vi "Use_Orig_XW_Stats.vi"() -> (5 "Plug in titles":string[](array[string]), 7 "Plug in values":string[](array[string]))   [LabVIEW 2010]
uses:
  Globals/Meas_global.vi
panel:
  in  "Invert 2nd Component?":bool
  out "Array":string[](array[string])
  in  "Template Filename":path=path "/G4_2_HD/Users/paulhayden/Projects/Hong Roughness/Reclaim data.tpt"
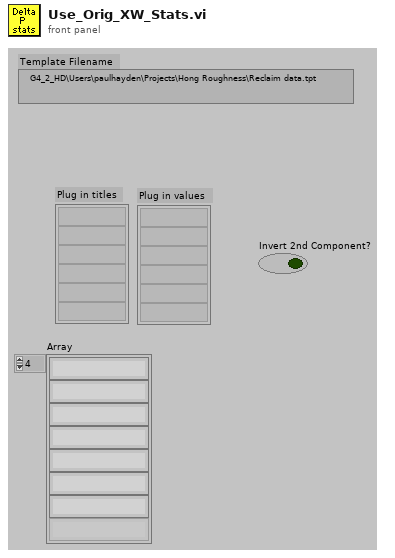
[diagram p1: front panel]
types:
  T1 = enum32{"existing file", "new file", "new or existing file", "existing dir", "new dir", "new or existing dir", "existing file (use LLBs)", "new file (use LLBs)", "new or existing file (use LLBs)", "new or existing file or directory (use LLBs)"}
  T2 = typedef "Analysis_type_cluster.ctl" = cluster{"Analysis type":T3, "Indicies":i32[], "Name":string, "Inst Array":T4, "Info index":i32}
  T3 = typedef "Analysis_type_Enum.ctl" = enum16{"Slow Response", "Fast Response", "Weighted Fast Response", "Fast FID", "Weighted Fast FID", "Cross Wire", "Weighted Cross Wire", "Weighted LDA"}
  T4 = typedef "Instrument_Array.ctl" = enum16{"PWA", "LDA", "Analogue"}
  T5 = typedef "Velocity_cluster.ctl" = cluster{"Name":string, "U":dbl, "u^2":dbl, "u^3/(u^2)^(1.5)":dbl, "u^4/(u^2)^2 -3":dbl, "% u'/U":dbl, "Mean % Err":dbl, "u^4":dbl}
  T6 = typedef "Correlation_cluster.ctl" = cluster{"U inst":string, "W inst":string, "uw":dbl, "uw/u'w'":dbl, "u^2w":dbl, "uw^2":dbl, "uw^3":dbl, "u^3w":dbl, "u^2w^2":dbl}
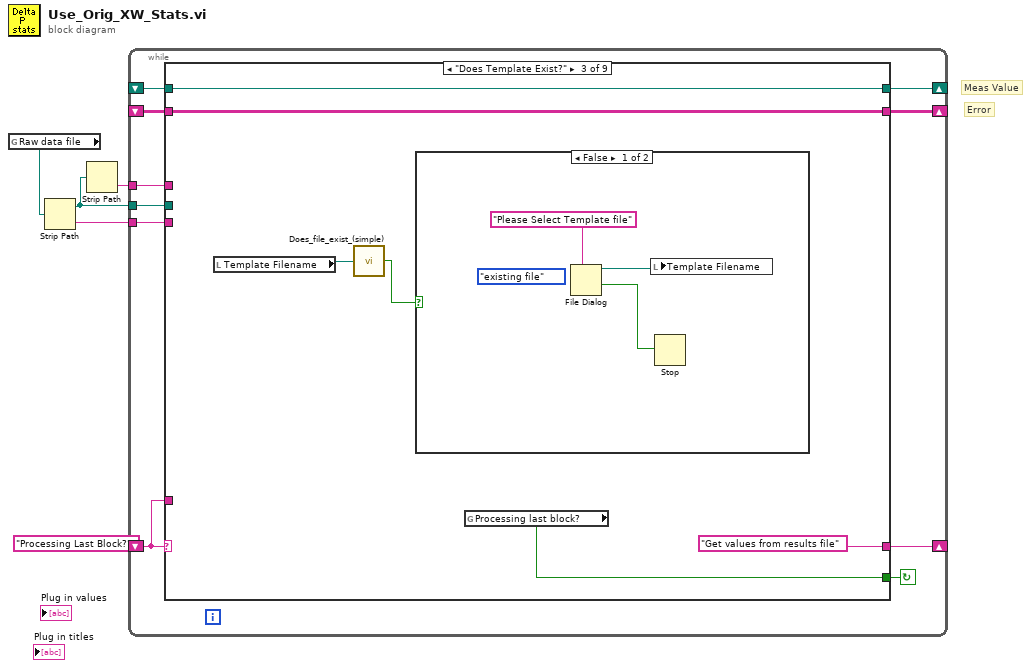
[diagram p0: block diagram]
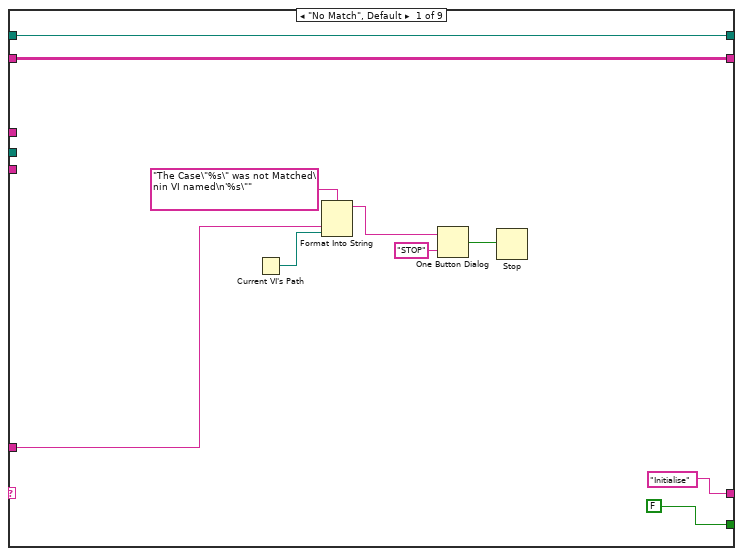
[diagram p2: hidden frame]
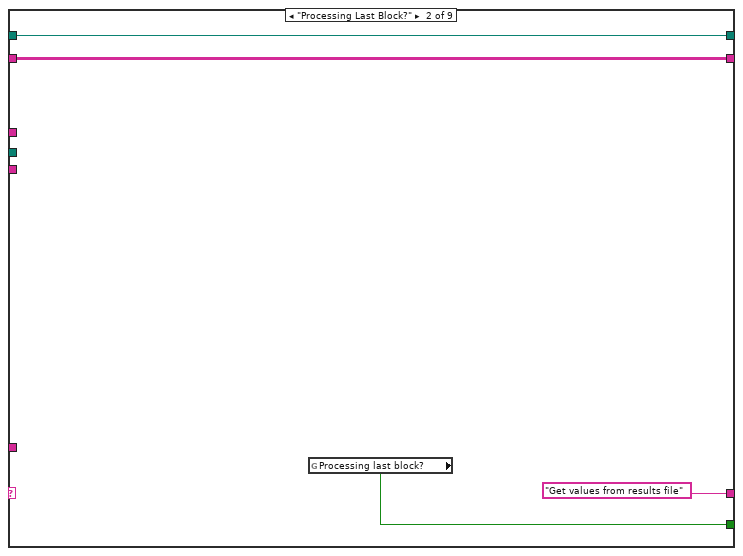
[diagram p3: hidden frame]
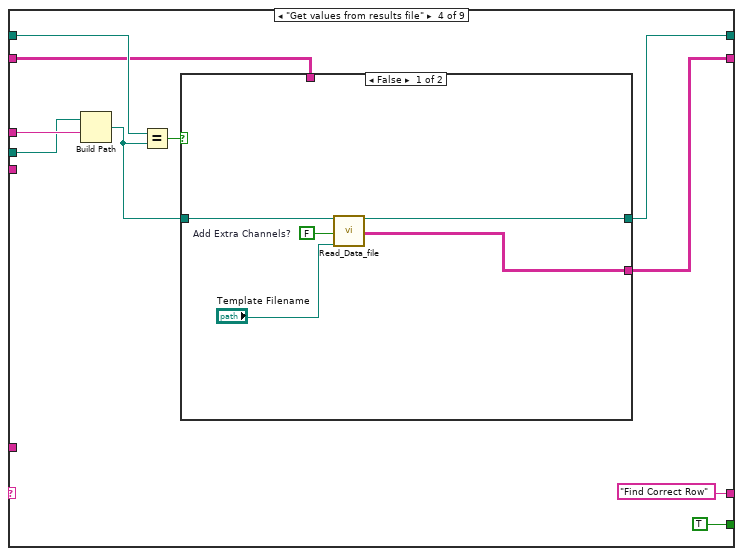
[diagram p5: hidden frame]
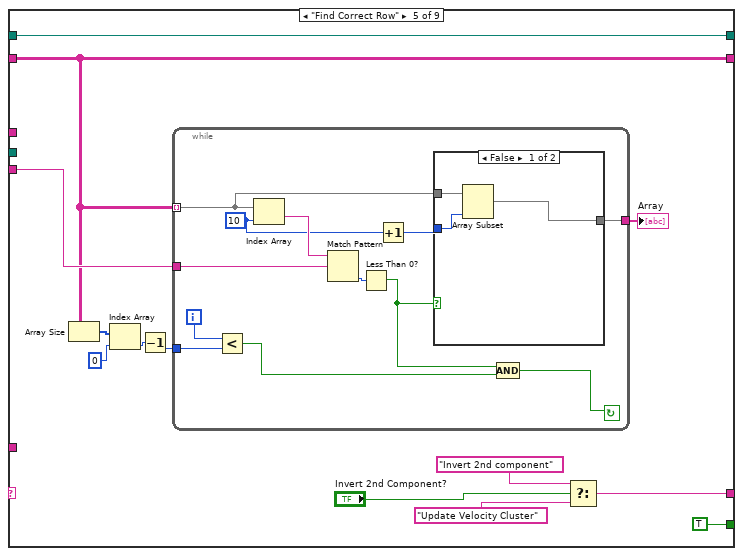
[diagram p7: hidden frame]
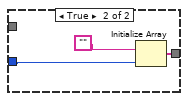
[diagram p8: hidden frame]
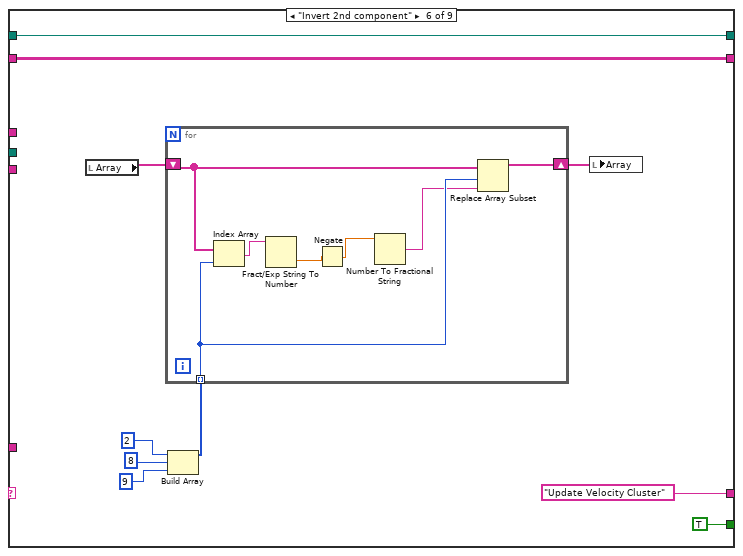
[diagram p9: hidden frame]
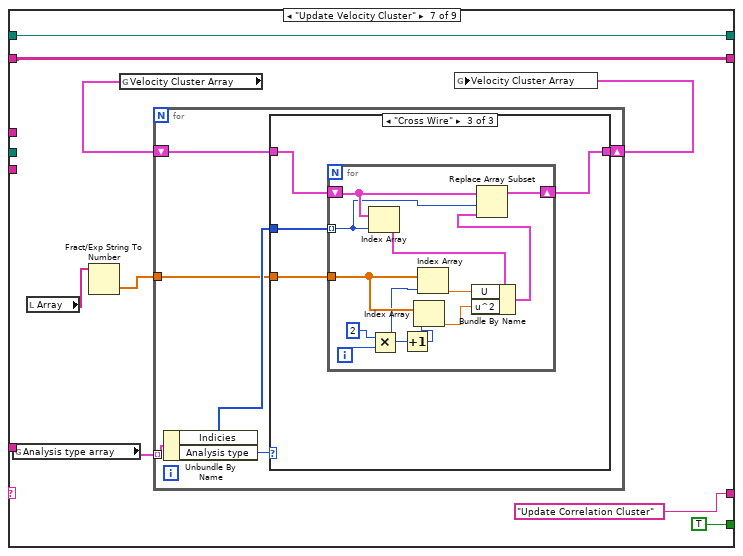
[diagram p10: hidden frame]
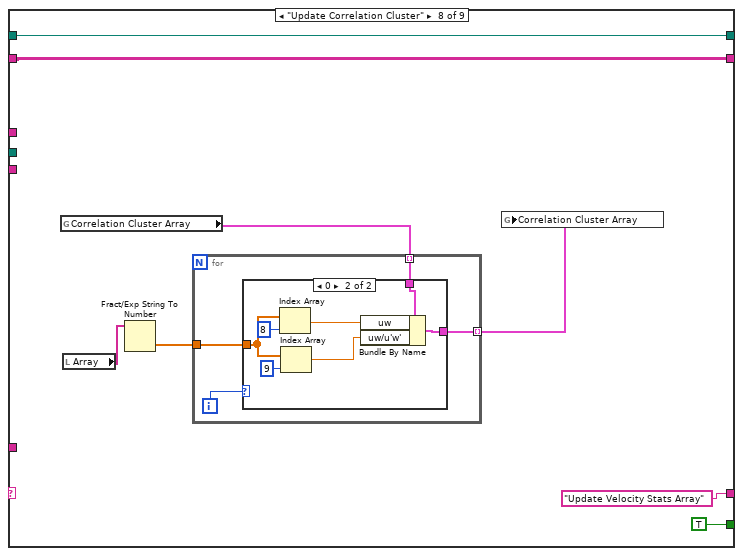
[diagram p13: hidden frame]
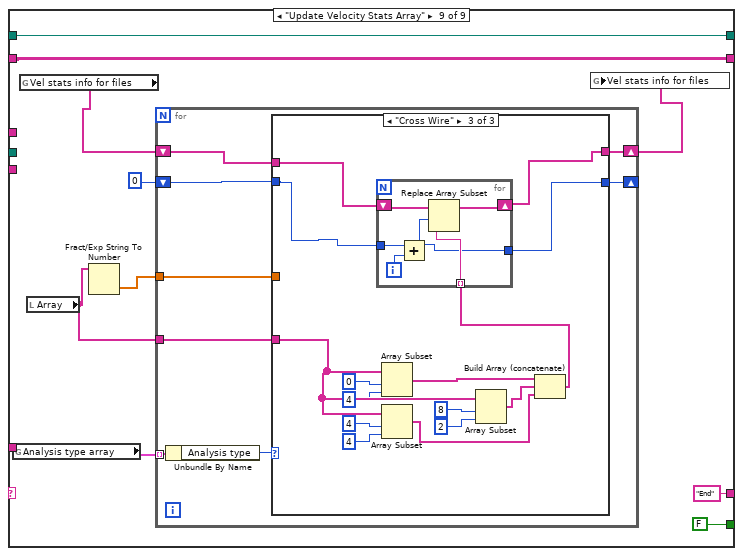
[diagram p15: hidden frame]
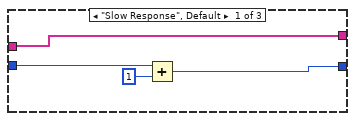
[diagram p16: hidden frame]
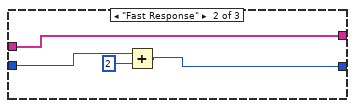
[diagram p17: hidden frame]
diagram:
  # "Error"
  # "Meas Value"
  n1 = global read "Meas_global.vi" "Raw data file"() -> (w4:path)
  n2 = Strip Path(path=w4) -> (stripped path=w2:path, name=w1:string)
  n3 = Strip Path(path=w2) -> (name=w3:string)  [unwired: 1 out]
  n4 = while {
    shift-left: _ -> [w9]
    shift-right: [w10] -> _
    shift-left: _ -> [w11]
    shift-right: [w12] -> _
    shift-left: "Processing Last Block?" -> [w13]
    shift-right: [w14] -> _
    tunnel: w3 -> [w8]
    tunnel: w2 -> [w7]
    tunnel: w1 -> [w6]
    stop <- w15 continue-if-true
    n5 = case shown="\"Does Template Exist?\"" w13 {
      tunnel: [FALSE w28 w34 TRUE ("Processing last block?") TRUE ("Processing last block?") TRUE ("Processing last block?") TRUE ("Processing last block?") TRUE ("Processing last block?") FALSE ("Processing last block?")] -> w15
      tunnel: ["Initialise" "Get values from results file" "Get values from results file" "Find Correct Row" w59 "Update Velocity Cluster" "Update Correlation Cluster" "Update Velocity Stats Array" "End"] -> w14
      tunnel: w13 -> [w20 _ _ _ _ _ _ _ _]
      tunnel: [w17 w27 w33 w39 w61 w96 w111 w143 w165] -> w12
      tunnel: w11 -> [w17 w27 w33 w42 w61 w96 w111 w143 w165]
      tunnel: [w16 w26 w32 w41 w62 w94 w109 w141 w163] -> w10
      tunnel: w9 -> [w16 w26 w32 w40 w62 w94 w109 w141 w163]
      tunnel: w8 -> [_ _ _ w46 _ _ _ _ _]
      tunnel: w7 -> [_ _ _ w45 _ _ _ _ _]
      tunnel: w6 -> [_ _ _ _ w68 _ _ _ _]
      frame "No Match", Default {
        n6 = Current VI's Path() -> (path=w19:path)
        n7 = Format Into String(format string="The Case\"%s\" was not Matched\nin VI named\n'%s\"" ("Format String"), w20, w19) -> (resulting string=w23:string)  [unwired: 2 in, 1 out]
        n8 = One Button Dialog(message=w23, button name ("OK")="STOP") -> (true=w21:bool)
        n9 = Stop(stop? (T)=w21) -> ()
      }
      frame "Processing Last Block?" {
        n10 = global read "Meas_global.vi" "Processing last block?"() -> (w28:bool)
      }
      frame "Does Template Exist?" {
        n11 = local read "Template Filename"() -> (w31:path)
        n12 = call "Does_file_exist_(simple).vi"("Pathname"=w31) -> ("exists?"=w30:bool)
        n13 = case shown="False" w30 {
          frame False {
            (unwired) T1."existing file" ("select mode (2)")
            n14 = File Dialog(7:"Please Select Template file" ("prompt")) -> (1:w36:bool, 3:w37:path)  [unwired: 1 in, 7 out]
            n15 = local write "Template Filename"(w37) -> ()
            n16 = Stop(stop? (T)=w36) -> ()
          }
          frame True {
          }
        }
        n17 = global read "Meas_global.vi" "Processing last block?"() -> (w34:bool)
      }
      frame "Get values from results file" {
        n18 = Build Path(base path=w45, name or relative path=w46) -> (appended path=w43:path)
        n19 = Equal?(x=w42, y=w43) -> (x = y?=w44:bool)
        n20 = case shown="False" w44 {
          tunnel: w43 -> [w51 w55]
          tunnel: [w50 w55] -> w39
          tunnel: [w49 w54] -> w41
          tunnel: w40 -> [_ w54]
          frame False {
            w52 = FALSE  # Add Extra Channels?
            n21 = call "Read_Data_file.vi"("Results file"=w51, "Add Extra Channels?"=w52, "Template File"="Template Filename") -> ("Results file Out"=w50:path, "Channel Values Out"=w49:string[][])  [unwired: 2 in, 13 out]
          }
          frame True {
          }
        }
      }
      frame "Find Correct Row" {
        n22 = Array Size(array=w62) -> (size(s)=w67:i32[])
        n23 = Index Array(array=w67, index=0) -> (element=w65:i32)
        n24 = Decrement(x=w65) -> (x-1=w64:i32)
        n25 = while {
          tunnel: w62 -> [w72] mode=indexing
          tunnel: w68 -> [w79]
          tunnel: w64 -> [w77]
          tunnel: [w71] -> w63
          i -> [w78]
          stop <- w74 continue-if-true
          w70 = 10 ("index")
          n26 = Less?(x=w78, y=w77) -> (x < y?=w75:bool)
          n27 = Index Array(array=w72, index=w70) -> (element=w80:string)
          n28 = Match Pattern(string=w80, regular expression=w79) -> (offset past match=w76:i32)  [unwired: 4 out]
          n29 = Less Than 0?(x=w76) -> (x < 0?=w73:bool)
          n30 = Increment(x=w70) -> (x+1=w69:i32)
          n31 = case shown="False" w73 {
            tunnel: w72 -> [w83 _]
            tunnel: [w81 w86] -> w71
            tunnel: w69 -> [w82 w85]
            frame False {
              n32 = Array Subset(array=w83, length=w82) -> (w81:string[])  [unwired: 1 in]
            }
            frame True {
              n33 = Initialize Array("", w85) -> (w86:string[])
            }
          }
          n34 = Compound Arithmetic op=AND(w73, w75) -> (w74:bool)
        }
        "Array" <- w63
        n35 = Select(t="Invert 2nd component" ("f"), s="Invert 2nd Component?", f="Update Velocity Cluster") -> (s? t:f=w59:string)
      }
      frame "Invert 2nd component" {
        n36 = local read "Array"() -> (w92:string[])
        n37 = Build Array(2, 8, 9) -> (w88:i32[])
        n38 = for {
          shift-right: [w103] -> w87
          shift-left: w92 -> [w102]
          tunnel: w88 -> [w101] mode=indexing
          n39 = Index Array(array=w102, index=w101) -> (element=w100:string)
          n40 = Fract/Exp String To Number(string=w100) -> (number=w99:dbl)  [unwired: 4 out]
          n41 = Negate(x=w99) -> (-x=w98:dbl)
          n42 = Number To Fractional String(number=w98) -> (F-format string=w97:string)  [unwired: 3 out]
          n43 = Replace Array Subset(array=w102, new element=w97, index=w101) -> (w103:string[])
        }
        n44 = local write "Array"(w87) -> ()
      }
      frame "Update Velocity Cluster" {
        n45 = global read "Meas_global.vi" "Analysis type array"() -> (w106:T2[])
        n46 = local read "Array"() -> (w104:string[])
        n47 = Fract/Exp String To Number(string=w104) -> (number=w105:dbl[])  [unwired: 4 out]
        n48 = global read "Meas_global.vi" "Velocity Cluster Array"() -> (w108:T5[])
        n49 = for {
          shift-right: [w115] -> w107
          shift-left: w108 -> [w116]
          tunnel: w106 -> [w118] mode=indexing
          tunnel: w105 -> [w113]
          n50 = Unbundle By Name(w118) -> ("Indicies"=w114:i32[], "Analysis type"=w117:T3)
          n51 = case shown="\"Cross Wire\"" w117 {
            tunnel: w116 -> [w119 w120 w124]
            tunnel: [w119 w120 w123] -> w115
            tunnel: w114 -> [_ _ w122]
            tunnel: w113 -> [_ _ w121]
            frame "Slow Response", Default {
            }
            frame "Fast Response" {
            }
            frame "Cross Wire" {
              n52 = for {
                shift-right: [w133] -> w123
                shift-left: w124 -> [w132]
                tunnel: w122 -> [w129] mode=indexing
                tunnel: w121 -> [w126]
                i -> [w136]
                n53 = Index Array(array=w132, index=w129) -> (element=w131:T5)
                n54 = Multiply(x=2, y=w136) -> (x*y=w125:i32)
                n55 = Increment(x=w125) -> (x+1=w134:i32)
                n56 = Index Array(array=w126, index=w134) -> (element=w127:dbl)
                n57 = Index Array(array=w126, index=w125) -> (element=w128:dbl)
                n58 = Bundle By Name(cluster=w131, "U"=w128, "u^2"=w127) -> (w130:T5)
                n59 = Replace Array Subset(array=w132, new element=w130, index=w129) -> (w133:T5[])
              }
            }
          }
        }
        n60 = global write "Meas_global.vi" "Velocity Cluster Array"(w107) -> ()
      }
      frame "Update Correlation Cluster" {
        n61 = global read "Meas_global.vi" "Correlation Cluster Array"() -> (w140:T6[])
        n62 = local read "Array"() -> (w139:string[])
        n63 = Fract/Exp String To Number(string=w139) -> (number=w138:dbl[])  [unwired: 4 out]
        n64 = for {
          tunnel: w140 -> [w148] mode=indexing
          tunnel: w138 -> [w147]
          tunnel: [w146] -> w137 mode=indexing
          i -> [w145]
          n65 = case shown="0" w145 {
            tunnel: w148 -> [w149 w156]
            tunnel: w147 -> [_ w155]
            tunnel: [w149 w150] -> w146
            frame 1, Default {
            }
            frame 0 {
              n66 = Index Array(array=w155, index=8) -> (element=w154:dbl)
              n67 = Index Array(array=w155, index=9) -> (element=w153:dbl)
              n68 = Bundle By Name(cluster=w156, "uw"=w154, "uw/u'w'"=w153) -> (w150:T6)
            }
          }
        }
        n69 = global write "Meas_global.vi" "Correlation Cluster Array"(w137) -> ()
      }
      frame "Update Velocity Stats Array" {
        n70 = global read "Meas_global.vi" "Analysis type array"() -> (w162:T2[])
        n71 = global read "Meas_global.vi" "Vel stats info for files"() -> (w158:string[])
        n72 = local read "Array"() -> (w160:string[])
        n73 = Fract/Exp String To Number(string=w160) -> (number=w161:dbl[])  [unwired: 4 out]
        n74 = for {
          tunnel: w162 -> [w174] mode=indexing
          tunnel: w161 -> [w172]
          tunnel: w160 -> [w171]
          shift-right: [w168] -> w159
          shift-left: w158 -> [w167]
          shift-right: [w169] -> _
          shift-left: 0 -> [w170]
          n75 = Unbundle By Name(w174) -> ("Analysis type"=w173:T3)
          n76 = case shown="\"Cross Wire\"" w173 {
            tunnel: [w178 w179 w193] -> w168
            tunnel: w172 -> [_ _ _]
            tunnel: w171 -> [_ _ w195]
            tunnel: w170 -> [w177 w182 w196]
            tunnel: [w175 w180 w194] -> w169
            tunnel: w167 -> [w178 w179 w197]
            frame "Slow Response", Default {
              n77 = Add(x=w177, y=1) -> (x+y=w175:i32)
            }
            frame "Fast Response" {
              n78 = Add(x=w182, y=2) -> (x+y=w180:i32)
            }
            frame "Cross Wire" {
              n79 = Array Subset(array=w195, index=0, length=4) -> (w188:string[])
              n80 = Array Subset(array=w195, index=4, length=4) -> (w184:string[])
              n81 = Array Subset(array=w195, index=8, length=2) -> (w185:string[])
              n82 = Build Array (concatenate)(w188, w185, w184) -> (w183:string[])
              n83 = for {
                shift-right: [w202] -> w193
                shift-left: w197 -> [w203]
                tunnel: w196 -> [w200]
                tunnel: w183 -> [w199] mode=indexing
                tunnel: [w198] -> w194
                i -> [w201]
                n84 = Add(x=w200, y=w201) -> (x+y=w198:i32)
                n85 = Replace Array Subset(array=w203, new element=w199, index=w198) -> (w202:string[])
              }
            }
          }
        }
        n86 = global write "Meas_global.vi" "Vel stats info for files"(w159) -> ()
      }
    }
  }
